vi "AlliGator Save Calibration Phasor.vi"(8 "Error In":errorcluster, 11 "Calibration Phasor":T1) -> (0 "error out":errorcluster, 1 "Message":string, 3 "XML File Path":path)   [LabVIEW 2021, in "AlliGator Phasor Calibration.lvlib"]
doc: "Saves the <B>Phasor Calibration</B>."
uses:
  AlliGator Phasor Calibration.lvlib
  Phasor/Calibration Phasor (m, phi).ctl
  Files/Files.lvlib
  Phasor/Phasor.lvlib
panel:
  # "see the AlliGator License on the block diagram (Ctrl+E or Window:Show Block Diagram)"
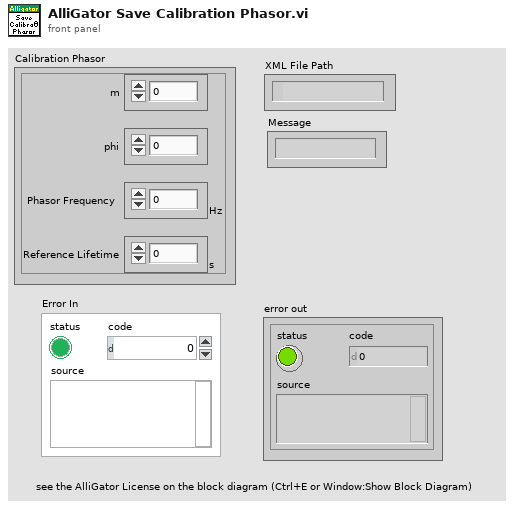
[diagram p1: front panel]
types:
  T1 = typedef "Phasor.lvlib/Calibration Phasor (m, phi).ctl" = cluster{"m":dbl, "phi":dbl, "Phasor Frequency":dbl[unit], "Reference Lifetime":dbl[unit]}
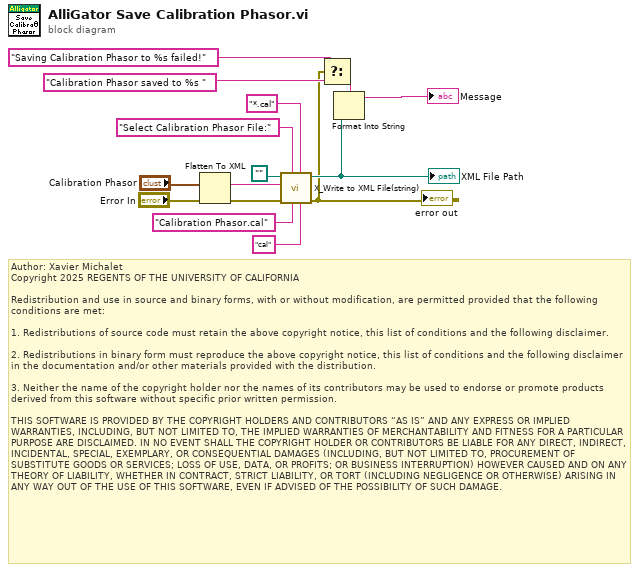
[diagram p0: block diagram]
diagram:
  # "Author: Xavier Michalet\nCopyright 2025 REGENTS OF THE UNIVERSITY OF CALIFORNIA\n\nRedistribution and use in source and binary forms, with or without modification, are permitted provided that the following conditions are met:\n\n1. Redistributions of source code must retain the above copyright notice, this list of conditions and the following disclaimer.\n\n2. Redistributions in binary form must reproduce the above copyright notice, this list of conditions and the following disclaimer in the documentation and/or other materials provided with the distribution.\n\n3. Neither the name of the copyright holder nor the names of its contributors may be used to endorse or promote products derived from this software without specific prior written permission.\n\nTHIS SOFTWARE IS PROVIDED BY THE COPYRIGHT HOLDERS AND CONTRIBUTORS “AS IS” AND ANY EXPRESS OR IMPLIED WARRANTIES, INCLUDING, BUT NOT LIMITED TO, THE IMPLIED WARRANTIES OF MERCHANTABILITY AND FITNESS FOR A PARTICULAR PURPOSE ARE DISCLAIMED. IN NO EVENT SHALL THE COPYRIGHT HOLDER OR CONTRIBUTORS BE LIABLE FOR ANY DIRECT, INDIRECT, INCIDENTAL, SPECIAL, EXEMPLARY, OR CONSEQUENTIAL DAMAGES (INCLUDING, BUT NOT LIMITED TO, PROCUREMENT OF SUBSTITUTE GOODS OR SERVICES; LOSS OF USE, DATA, OR PROFITS; OR BUSINESS INTERRUPTION) HOWEVER CAUSED AND ON ANY THEORY OF LIABILITY, WHETHER IN CONTRACT, STRICT LIABILITY, OR TORT (INCLUDING NEGLIGENCE OR OTHERWISE) ARISING IN ANY WAY OUT OF THE USE OF THIS SOFTWARE, EVEN IF ADVISED OF THE POSSIBILITY OF SUCH DAMAGE."
  n1 = Flatten To XML(6:"Calibration Phasor") -> (2:w13:string)
  n2 = call "X_Write to XML File(string).vi"("File Extension (xml)"="cal", "Pattern (*.xml;*.XML)"="*.cal", "default name"="Calibration Phasor.cal", "Prompt"="Select Calibration Phasor File:", "error in (no error)"="Error In", "XML Input"=w13, "XML File Start Path"=path "") -> ("error out"=w3:errorcluster, "XML File Path"=w12:path)  [unwired: 1 in, 2 out]
  "XML File Path" <- w12
  "error out" <- w3
  n3 = Select(t="Saving Calibration Phasor to %s failed!" ("format string"), s=w3, f="Calibration Phasor saved to %s " ("format string")) -> (s? t:f=w11:string)
  n4 = Format Into String(format string=w11, w12) -> (resulting string=→"Message":string)  [unwired: 2 in, 1 out]
